vi "CRC-16-2.vi"(11 "U8":u8[](array[numeric]) format="%.0x") -> (3 "CRC-16":u16 format="%.0x")   [LabVIEW 2019]
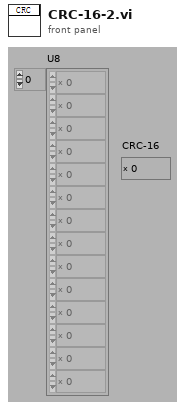
[diagram p1: front panel]
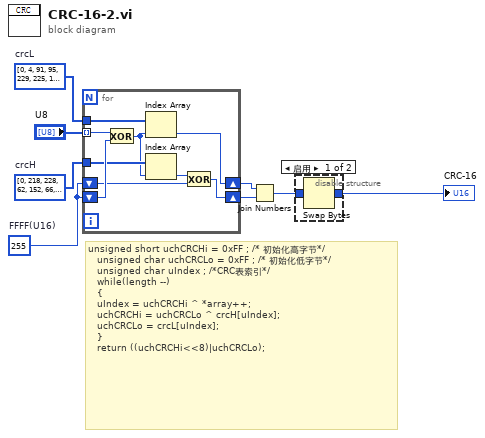
[diagram p0: block diagram]
diagram:
  w4 = u8[] [0, 4, 91, 95, 229, 225, 190, 186, 153, 157, 194, 198, 124, 120, 39, 35, 50, 54, 105, 109, 215, 211, 140, 136, 171, 175, 240, 244, 78, 74, 21, 17, 55, 51, 108, 104, 210, 214, 137, 141, 174, 170, 245, 241, 75, 79, 16, 20, 5, 1, 94, 90, 224, 228, 187, 191, 156, 152, 199, 195, 121, 125, 34, 38, 61, 57, 102, 98, 216, 220, 131, 135, 164, 160, 255, 251, 65, 69, 26, 30, 15, 11, 84, 80, 234, 238, 177, 181, 150, 146, 205, 201, 115, 119, 40, 44, 10, 14, 81, 85, 239, 235, 180, 176, 147, 151, 200, 204, 118, 114, 45, 41, 56, 60, 99, 103, 221, 217, 134, 130, 161, 165, 250, 254, 68, 64, 31, 27, 41, 45, 114, 118, 204, 200, 151, 147, 176, 180, 235, 239, 85, 81, 14, 10, 27, 31, 64, 68, 254, 250, 165, 161, 130, 134, 217, 221, 103, 99, 60, 56, 30, 26, 69, 65, 251, 255, 160, 164, 135, 131, 220, 216, 98, 102, 57, 61, 44, 40, 119, 115, 201, 205, 146, 150, 181, 177, 238, 234, 80, 84, 11, 15, 20, 16, 79, 75, 241, 245, 170, 174, 141, 137, 214, 210, 104, 108, 51, 55, 38, 34, 125, 121, 195, 199, 152, 156, 191, 187, 228, 224, 90, 94, 1, 5, 35, 39, 120, 124, 198, 194, 157, 153, 186, 190, 225, 229, 95, 91, 4, 0, 17, 21, 74, 78, 244, 240, 175, 171, 136, 140, 211, 215, 109, 105, 54, 50]  # crcL
  w5 = u8[] [0, 218, 228, 62, 152, 66, 124, 166, 97, 187, 133, 95, 249, 35, 29, 199, 195, 25, 39, 253, 91, 129, 191, 101, 162, 120, 70, 156, 58, 224, 222, 4, 214, 12, 50, 232, 78, 148, 170, 112, 183, 109, 83, 137, 47, 245, 203, 17, 21, 207, 241, 43, 141, 87, 105, 179, 116, 174, 144, 74, 236, 54, 8, 210, 252, 38, 24, 194, 100, 190, 128, 90, 157, 71, 121, 163, 5, 223, 225, 59, 63, 229, 219, 1, 167, 125, 67, 153, 94, 132, 186, 96, 198, 28, 34, 248, 42, 240, 206, 20, 178, 104, 86, 140, 75, 145, 175, 117, 211, 9, 55, 237, 233, 51, 13, 215, 113, 171, 149, 79, 136, 82, 108, 182, 16, 202, 244, 46, 168, 114, 76, 150, 48, 234, 212, 14, 201, 19, 45, 247, 81, 139, 181, 111, 107, 177, 143, 85, 243, 41, 23, 205, 10, 208, 238, 52, 146, 72, 118, 172, 126, 164, 154, 64, 230, 60, 2, 216, 31, 197, 251, 33, 135, 93, 99, 185, 189, 103, 89, 131, 37, 255, 193, 27, 220, 6, 56, 226, 68, 158, 160, 122, 84, 142, 176, 106, 204, 22, 40, 242, 53, 239, 209, 11, 173, 119, 73, 147, 151, 77, 115, 169, 15, 213, 235, 49, 246, 44, 18, 200, 110, 180, 138, 80, 130, 88, 102, 188, 26, 192, 254, 36, 227, 57, 7, 221, 123, 161, 159, 69, 65, 155, 165, 127, 217, 3, 61, 231, 32, 250, 196, 30, 184, 98, 92, 134]  # crcH
  w7 = u8 255  # FFFF(U16)
  # "unsigned short uchCRCHi = 0xFF ; /* 初始化高字节*/\n\t  unsigned char uchCRCLo = 0xFF ; /* 初始化低字节*/\n\t  unsigned char uIndex ; /*CRC表索引*/\n\t  while(length --)\n\t  {\n\t\t uIndex = uchCRCHi ^ *array++;\n\t\t uchCRCHi = uchCRCLo ^ crcH[uIndex];\n\t\t uchCRCLo = crcL[uIndex];\n\t  }\n\t  return ((uchCRCHi<<8)|uchCRCLo);"
  n1 = for {
    tunnel: "U8" -> [w16] mode=indexing
    tunnel: w5 -> [w15]
    tunnel: w4 -> [w14]
    shift-right: [w10] -> w3
    shift-left: w7 -> [w9]
    shift-right: [w11] -> w2
    shift-left: w7 -> [w17]
    n2 = Exclusive Or(1:w17, 2:w16) -> (0:w13:u8)
    n3 = Index Array(array=w14, index=w13) -> (element=w10:u8)
    n4 = Index Array(array=w15, index=w13) -> (element=w12:u8)
    n5 = Exclusive Or(1:w9, 2:w12) -> (0:w11:u8)
  }
  n6 = Join Numbers(hi=w3, lo=w2) -> ((hi.lo)=w8:u16)
  n7 = disable-structure shown="启用" {
    disable-tunnel: w8 -> [w19 w20]
    disable-tunnel: [w18 w20] -> w1
    frame Enabled {
      n8 = Swap Bytes(anything=w19) -> (byte swapped=w18:u16)
    }
    frame Disabled {
    }
  }
  "CRC-16" <- w1
